vi "python simple example.vi"() -> ()   [LabVIEW 2018]
panel:
  in  "# loops":i32=1
  out "time per":dbl=2.0
  in  "open h5":string="test"
  out "return string time":u32=2
  out "open session time":u32=247
  in  "par":string="poop"
  in  "Python version":string="3.8"
  out "return value":string="poop"
  in  "function name":string="test"
  in  "module path":path=path "C:/Users/tony_/Downloads/2020_04_24_PNG_HDF5_Benchmark_Tony/2020_04_24_PNG_HDF5_Benchmark_Tony/testmodule.py"
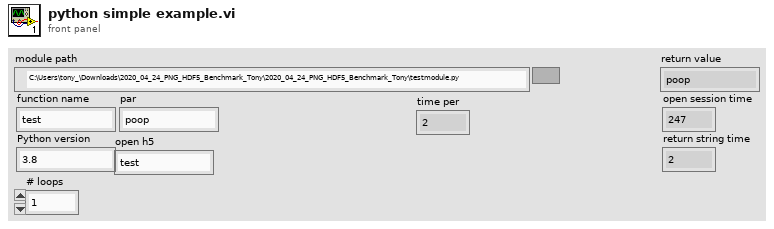
[diagram p1: front panel]
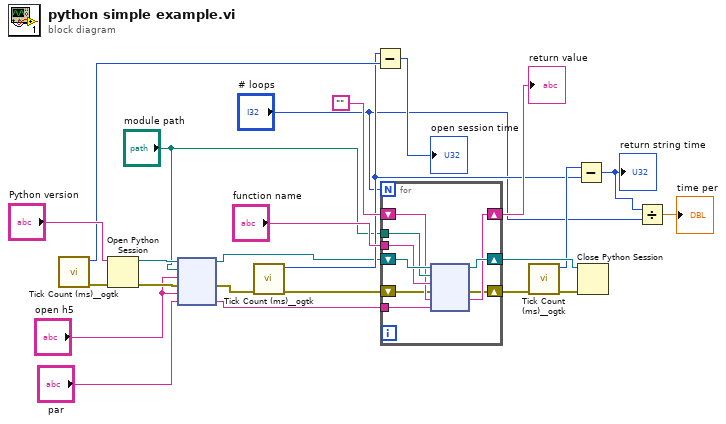
[diagram p0: block diagram]
diagram:
  n1 = call <userlib>:"Tick Count (ms)__ogtk.vi"() -> ("error out"=w18:errorcluster, "millisecond timer value"=w19:u32)  [unwired: 10 in]
  n2 = Open Python Session(python version="Python version", 3:w18) -> (session out=w11:refnum<k35>, error out=w10:errorcluster)  [unwired: 1 in]
  n3 = node(w11, "module path", "open h5", w10, "open h5", "par") -> (w8:refnum<k35>, w7:errorcluster, w4:string)  [unwired: 1 in, 2 out]
  n4 = call <userlib>:"Tick Count (ms)__ogtk.vi"("error in (no error)"=w7) -> ("error out"=w17:errorcluster, "millisecond timer value"=w13:u32)  [unwired: 9 in]
  n5 = Subtract(x=w13, y=w19) -> (x-y=→"open session time":u32)
  n6 = for {
    N: "# loops" -> [_]
    tunnel: "module path" -> [w31]
    tunnel: "function name" -> [w30]
    tunnel: w4 -> [w27]
    shift-right: [w32] -> w23
    shift-left: w8 -> [w33]
    shift-right: [w28] -> w20
    shift-left: "" -> [w29]
    shift-right: [w25] -> w16
    shift-left: w17 -> [w26]
    n7 = node(w33, w31, w30, w26, w29, w27) -> (w32:refnum<k35>, w25:errorcluster, w28:string)  [unwired: 1 in, 2 out]
  }
  "return value" <- w20
  n8 = call <userlib>:"Tick Count (ms)__ogtk.vi"("error in (no error)"=w16) -> ("error out"=w15:errorcluster, "millisecond timer value"=w14:u32)  [unwired: 9 in]
  n9 = Subtract(x=w14, y=w13) -> (x-y=w3:u32)
  "return string time" <- w3
  n10 = Close Python Session(session in=w23, error in=w15) -> ()  [unwired: 1 out]
  n11 = Divide(x=w3, y="# loops") -> (x/y=→"time per":dbl)
